vi "Phasor Explorer Settings Window.vi"() -> ()   [LabVIEW 2019]
uses:
  Phasor Explorer Detector Parameters.ctl
  Phasor Explorer Gate Parameter to Adjust.ctl
  Phasor Explorer Gate Parameters.ctl
  Gate Type.ctl
  Type of User-defined Function.ctl
  Phasor Explorer Decay Parameters.ctl
  IRF Model.ctl
  Phasor Explorer Phasor Parameters.ctl
  Phasor Calculation Type.ctl
  SEPL Type.ctl
  Phasor Explorer Display Parameters.ctl
  Type of Series.ctl
  Phasor Explorer Q [Element].ctl
  Phasor Explorer Q [Event] List.ctl
panel:
  in  "Parameter Tabs":T1(tab)=enum."Gates"
  in  "Display Parameters":T2={"# Points"=1000, "Ramp Type"=enum."Logarithmic", "Type of Series"=enum."1-Exp Decays", "Min tau"=1.0000000000000002e-12, "Max tau"=1.0000000000000001e-07, "Include 0"=FALSE, "Include Infinity"=FALSE} {"Min tau" min=0.0; "Max tau" min=0.0; "# Points" min=1 step=1}
  out "f*":dbl[unit]=80000000.0 format="%#_5g"
  out "tau*":dbl[unit]=1.9894367886486918e-09 format="%#_5g"
  in  "Phasor Parameters":T4={"Harmonic Frequency"=80000000.0, "Use f* = 1/D Frequency"=FALSE, "Calibrated Phasor"=FALSE, "Calibration Lifetime"=1e-09, "Phasor Calculation"=enum."Direct Sum", "SEPL Type"=enum."UC", "# Gates"=1.0, "Square Gate Width"=1e-09, "Show Ticks"=FALSE} {"Square Gate Width" min=0.0; "# Gates" min=0.0; "Calibration Lifetime" min=0.0; "Harmonic Frequency" min=0.0}
  in  "Decay & IRF Parameters":T7={"Lifetime"=3.0000000000000004e-09, "IRF Offset"=0.0, "IRF Period"=1.2500000000000001e-08, "Normalized Decays"=FALSE, "IRF Model"=enum."Dirac", "IRF Parameter 1"=0.0} {"Lifetime" min=0.0; "IRF Period" min=0.0}
  in  "Edit User-defined Gate":bool
  in  "Gate Parameter to Adjust":T9 caption="Adjust"
  in  "Match Laser Period":bool=TRUE
  in  "Gate Parameters":T10={"First Gate Start"=0.0, "Use Gate Center"=FALSE, "Gate Width"=0.0, "Gate Step"=1.785714285714286e-09, "# Gates"=7.0, "Gate Type"=enum."Square", "Edge Width"=0.0, "Top Slope"=0.0, "Reversed Sawtooth?"=FALSE, "Analytical Computation"=FALSE, "Integration"=enum."Item 0", "Tolerance"=1.0, "# Steps"=1.0, "Type of User-defined Function"=enum."Gate", "Use Gate Step"=FALSE} caption="Phasor Explorer Gate Parameters" {"# Steps" min=0.0; "Tolerance" min=0.0; "Top Slope" min=0.0; "Edge Width" min=0.0; "Gate Step" min=0.0; "# Gates" min=1.0 step=1.0; "Gate Width" min=0.0}
  in  "Detector Parameters":T13={"Frames/Image"=0, "Gates/Frame"=1, "Bits/Frame"=1, "Multiplicity"=0, "Incident Signal"=0.0, "Poisson Signal"=FALSE} {"Frames/Image" min=1; "Multiplicity" min=0; "Bits/Frame" min=1; "Gates/Frame" min=1}
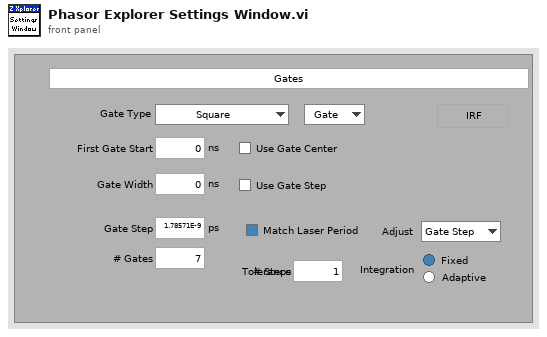
[diagram p1: front panel]
types:
  T1 = enum32{"Display", "Phasor", "Decay", "Gates", "Detector"}
  T2 = typedef "Phasor Explorer Display Parameters.ctl" = cluster{"# Points":i32, "Ramp Type":enum16{"Linear", "Logarithmic"}, "Type of Series":T3, "Min tau":dbl[unit], "Max tau":dbl[unit], "Include 0":bool, "Include Infinity":bool}
  T3 = typedef "Type of Series.ctl" = enum16{"1-Exp Decays", "Linear Combination of 1-Exp"}
  T4 = typedef "Phasor Explorer Phasor Parameters.ctl" = cluster{"Harmonic Frequency":dbl[unit], "Use f* = 1/D Frequency":bool, "Calibrated Phasor":bool, "Calibration Lifetime":dbl[unit], "Phasor Calculation":T5, "SEPL Type":T6, "# Gates":dbl, "Square Gate Width":dbl[unit], "Show Ticks":bool}
  T5 = typedef "Phasor Calculation Type.ctl" = enum16{"Direct Sum", "Analytical Formula"}
  T6 = typedef "SEPL Type.ctl" = enum16{"UC", "L_N", "L_N[W]", "L_X"}
  T7 = typedef "Phasor Explorer Decay Parameters.ctl" = cluster{"Lifetime":dbl[unit], "IRF Offset":dbl[unit], "IRF Period":dbl[unit], "Normalized Decays":bool, "IRF Model":T8, "IRF Parameter 1":dbl[unit]}
  T8 = typedef "IRF Model.ctl" = enum16{"Dirac", "Exponential"}
  T9 = typedef "Phasor Explorer Gate Parameter to Adjust.ctl" = enum16{"Gate Step", "# Gates"}
  T10 = typedef "Phasor Explorer Gate Parameters.ctl" = cluster{"First Gate Start":dbl[unit], "Use Gate Center":bool, "Gate Width":dbl[unit], "Gate Step":dbl[unit], "# Gates":dbl, "Gate Type":T11, "Edge Width":dbl[unit], "Top Slope":dbl[unit], "Reversed Sawtooth?":bool, "Analytical Computation":bool, "Integration":enum32{"Item 0", "Item 1"}, "Tolerance":dbl, "# Steps":dbl, "Type of User-defined Function":T12, "Use Gate Step":bool}
  T11 = typedef "Gate Type.ctl" = enum16{"Square", "Finite Edge Square", "Finite Edge, Tilted Top Square", "Triangle", "Sawtooth", "User-defined"}
  T12 = typedef "Type of User-defined Function.ctl" = enum16{"Gate", "IRF"}
  T13 = typedef "Phasor Explorer Detector Parameters.ctl" = cluster{"Frames/Image":i32, "Gates/Frame":i32, "Bits/Frame":i32, "Multiplicity":i32, "Incident Signal":dbl, "Poisson Signal":bool}
  T14 = typedef "Phasor Explorer Q [Element].ctl" = cluster{"ZXP Q Event":T15, "Data":variant}
  T15 = typedef "Phasor Explorer Q [Event] List.ctl" = enum16{"Idle", "Initialization", "Show-Hide UC Ticks", "Edit User-defined Gate/IRF", "Update Phasor Graph", "Update Sum of Gates Graph", "Update Parameters", "Compute Decay &/or Gates", "Find Pseudo UC Intersections", "Compute alpha(beta) Plot", "Compute Pseudo-Phase Lifetime Plot", "Export Parameters to Clipboard", "Update Phase & Modulus Lifetime", "XY Graph Special Event", "Update Graph Plots Info", "Fit to Circle", "Quit"}
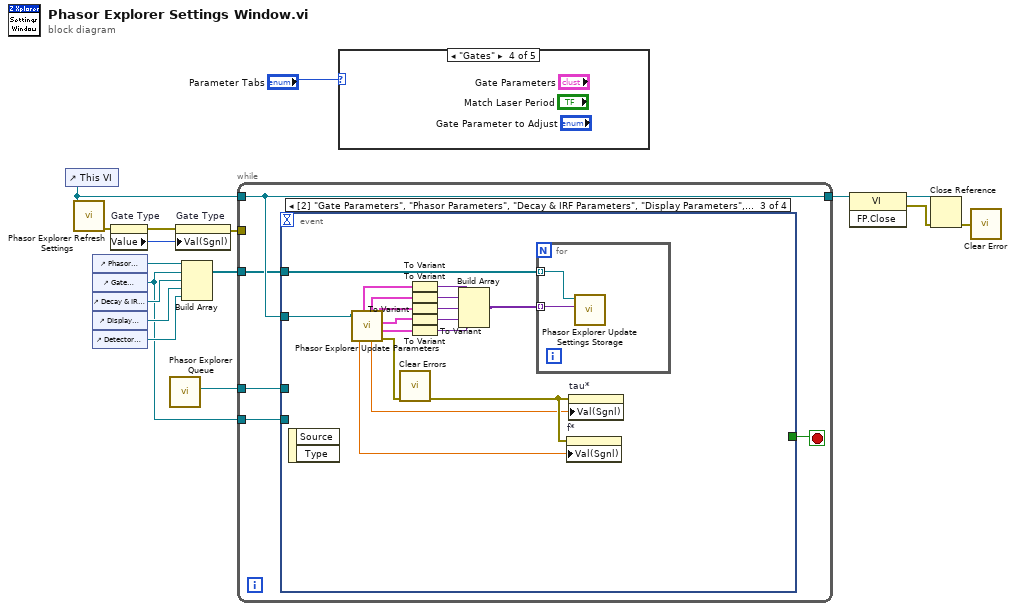
[diagram p0: block diagram]
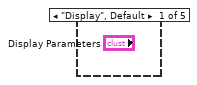
[diagram p2: hidden frame]
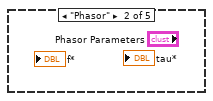
[diagram p3: hidden frame]
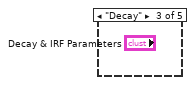
[diagram p4: hidden frame]
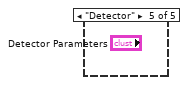
[diagram p5: hidden frame]
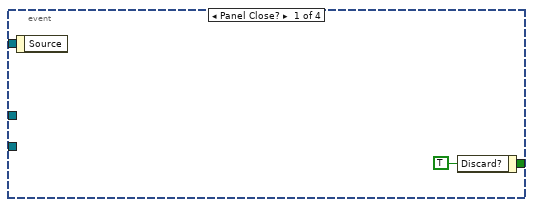
[diagram p6: hidden frame]
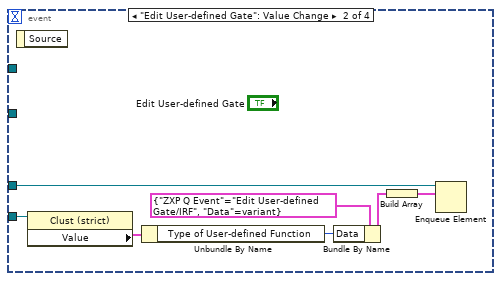
[diagram p7: hidden frame]
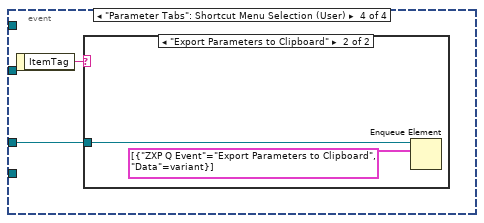
[diagram p8: hidden frame]
diagram:
  n1 = control-ref of="This VI"() -> (w10:refnum<vi>)
  n2 = call "Phasor Explorer Refresh Settings.vi"("VI in"=w10) -> ("error out"=w8:errorcluster)  [unwired: 10 in]
  n3 = control-ref of="Phasor Parameters"() -> (w6:refnum<vi>)
  n4 = control-ref of="Gate Parameters"() -> (w1:refnum<vi>)
  n5 = control-ref of="Decay & IRF Parameters"() -> (w4:refnum<vi>)
  n6 = control-ref of="Display Parameters"() -> (w3:refnum<vi>)
  n7 = control-ref of="Detector Parameters"() -> (w5:refnum<vi>)
  n8 = property on="Gate Type" class="Enum (strict)"(error in=w8) -> (error out=w11:errorcluster, "Value"=w14:T11)  [unwired: 1 in, 1 out]
  n9 = call "Phasor Explorer Queue.vi"() -> ("Phasor Explorer Queue"=w15:refnum<queue>)  [unwired: 11 in]
  n10 = property on="Gate Type" class="Enum (strict)"(error in=w11, "Val(Sgnl)"=w14) -> (error out=w9:errorcluster)  [unwired: 1 in, 1 out]
  n11 = Build Array(w6, w1, w4, w3, w5) -> (w2:refnum<vi>[])
  n12 = while {
    tunnel: [w21] -> w17
    tunnel: w9 -> [_]
    tunnel: w15 -> [w20]
    tunnel: w10 -> [w21]
    tunnel: w2 -> [w19]
    tunnel: w1 -> [w18]
    stop <- w22 stop-if-true
    n13 = event shown="[2] \"Gate Parameters\", \"Phasor Parameters\", \"Decay & IRF Parameters\", \"Display Parameters\", \"Match Laser Period\", \"Detector Parameters\": Value Change" {
      selector: _ -> [_ _ _ _]
      dyn-events: _ -> [_ _ _ _]
      timeout: _ -> [_ _ _ _]
      tunnel: [w23 _ _ _] -> w22
      tunnel: w21 -> [_ _ w47 _]
      tunnel: w20 -> [_ w30 _ w50]
      tunnel: w19 -> [_ _ w31 _]
      tunnel: w18 -> [_ w26 _ _]
      event Panel Close? {
        w23 = TRUE ("Discard?")
        n14 = event-data() -> ()  [unwired: 1 in, 1 out]
        n15 = event-data("Discard?"=w23) -> ()  [unwired: 1 in, 1 out]
      }
      event "Edit User-defined Gate": Value Change {
        n16 = event-data() -> ()  [unwired: 1 in, 1 out]
        n17 = property class="Clust (strict)"(reference=w26) -> ("Value"=w25:T10)  [unwired: 1 in, 2 out]
        n18 = Unbundle By Name(w25) -> ("Type of User-defined Function"=w24:T12)
        n19 = Bundle By Name(cluster=T14 {"ZXP Q Event"=enum."Edit User-defined Gate/IRF", "Data"=variant} ("element"), "Data"=w24) -> (w28:T14)
        n20 = Build Array(w28) -> (w27:T14[])
        n21 = Enqueue Element(queue=w30, element=w27) -> ()  [unwired: 2 in, 3 out]
      }
      event "Match Laser Period": Value Change {
        n22 = event-data() -> ()  [unwired: 1 in, 2 out]
        n23 = call "Phasor Explorer Update Parameters.vi"("VI in"=w47) -> ("error out"=w46:errorcluster, "Detector Parameters"=w38:T13, "Display Parameters"=w39:T2, "Decay & IRF Parameters"=w40:T7, "tau*"=w43:dbl[unit], "Gate Parameters"=w41:T10, "f0"=w44:dbl[unit], "Phasor Parameters"=w42:T4)  [unwired: 3 in]
        n24 = call <vilib>:"Clear Errors.vi"("error in (no error)"=w46) -> ("error out"=w45:errorcluster)  [unwired: 5 in, 1 out]
        n25 = To Variant(anything=w42) -> (Variant=w35:variant)
        n26 = To Variant(anything=w41) -> (Variant=w36:variant)
        n27 = To Variant(anything=w40) -> (Variant=w37:variant)
        n28 = To Variant(anything=w39) -> (Variant=w34:variant)
        n29 = To Variant(anything=w38) -> (Variant=w33:variant)
        n30 = Build Array(w35, w36, w37, w34, w33) -> (w32:variant[])
        n31 = for {
          tunnel: w32 -> [w49] mode=indexing
          tunnel: w31 -> [w48] mode=indexing
          n32 = call "Phasor Explorer Update Settings Storage.vi"("NewVal"=w49, "CtlRef"=w48) -> ()  [unwired: 9 in, 1 out]
        }
        n33 = property on="f*" class="DigNum (strict)"(error in=w45, "Val(Sgnl)"=w44) -> ()  [unwired: 1 in, 2 out]
        n34 = property on="tau*" class="DigNum (strict)"(error in=w45, "Val(Sgnl)"=w43) -> ()  [unwired: 1 in, 2 out]
      }
      event "Parameter Tabs": Shortcut Menu Selection (User) {
        n35 = event-data() -> ("ItemTag"=w51:string)  [unwired: 1 in]
        n36 = case shown="\"Export Parameters to Clipboard\"" w51 {
          tunnel: w50 -> [_ w53]
          frame "", Default {
          }
          frame "Export Parameters to Clipboard" {
            n37 = Enqueue Element(queue=w53, element=T14[] [{"ZXP Q Event"=enum."Export Parameters to Clipboard", "Data"=variant}]) -> ()  [unwired: 2 in, 3 out]
          }
        }
      }
    }
  }
  n38 = case shown="\"Gates\"" "Parameter Tabs" {
    frame "Display", Default {
    }
    frame "Phasor" {
    }
    frame "Decay" {
    }
    frame "Gates" {
    }
    frame "Detector" {
    }
  }
  n39 = invoke class="VI" method="FP.Close"(reference=w17) -> (reference out=w16:refnum<vi>, error out=w13:errorcluster)  [unwired: 2 in, 1 out]
  n40 = Close Reference(reference=w16, error in (no error)=w13) -> (error out=w12:errorcluster)
  n41 = call "Clear Error.vi"("Error In"=w12) -> ()  [unwired: 8 in, 1 out]
